vi "Set Selected Text Align.vi"(8 "error in (no error)":errorcluster caption="错误输入（无错误）", 10 "SelectionAlignment":i32(ring) items=["Left", "Right", "Center"], 11 "RichText 输入":refnum<class "RichText.lvclass"> caption="DNL_LabVIEW Object in") -> (0 "error out":errorcluster caption="错误输出", 3 "RichText 输出":refnum<class "RichText.lvclass"> caption="DNL_LabVIEW Object out")   [LabVIEW 2012, in "RichText.lvclass"]
uses:
  RichText.lvclass
  RichText.lvclass/RichText.ctl
  System.Windows.Forms
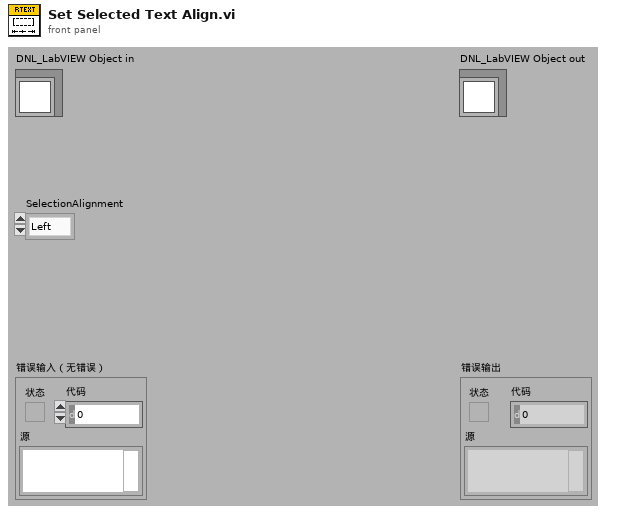
[diagram p1: front panel]
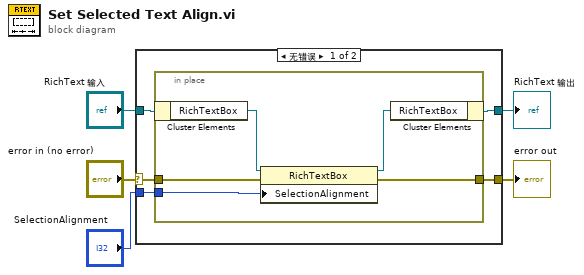
[diagram p0: block diagram]
diagram:
  n1 = case shown="无错误" "error in (no error)" {
    selector: "error in (no error)" -> [w9 w17]
    tunnel: [w7 w17] -> w4
    tunnel: [w8 w16] -> w2
    tunnel: "RichText 输入" -> [w10 w16]
    tunnel: "SelectionAlignment" -> [w6 _]
    frame No Error {
      n2 = in-place {
        in-place-border: w9 -> [w13]
        in-place-border: [w12] -> w7
        in-place-border: w6 -> [w11]
        n3 = in-place-cluster #1(w10) -> ("RichTextBox"=w15:refnum<k24>)
        n4 = property class="RichTextBox"(reference=w15, error in=w13, "SelectionAlignment"=w11) -> (reference out=w14:refnum<k24>, error out=w12:errorcluster)
        n5 = in-place-cluster #1("RichTextBox"=w14) -> (w8:refnum<class "RichText.lvclass">)
      }
    }
    frame Error {
    }
  }
  "error out" <- w4
  "RichText 输出" <- w2
